vi "ReadDigitalLine.vi"(0 "device name":string="DAQ", 5 "port":i32, 7 "line":i32, 11 "error in":errorcluster) -> (4 "state":u8, 15 "error out":errorcluster)   [LabVIEW 2012]
uses:
  <vilib>/DAQmx/read.llb/DAQmx Read.vi
  <vilib>/DAQmx/read.llb/DAQmx Read (Digital Bool 1Line 1Point).vi
  <vilib>/DAQmx/create/channels.llb/DAQmx Create Channel (DI-Digital Input).vi
  <vilib>/DAQmx/miscellaneous.llb/DAQmx Fill In Error Info.vi
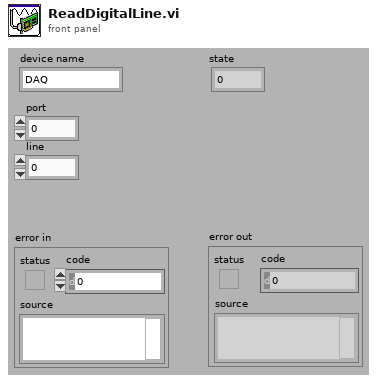
[diagram p1: front panel]
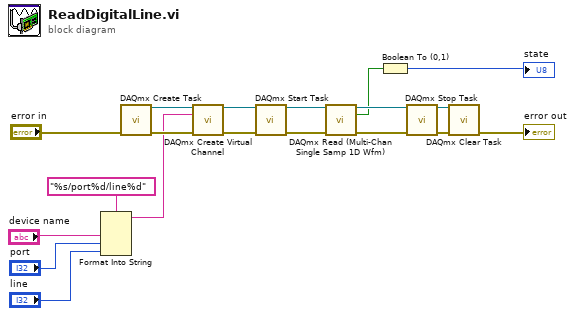
[diagram p0: block diagram]
diagram:
  n1 = Format Into String(format string="%s/port%d/line%d", "device name", "port", "line") -> (resulting string=w3:string)  [unwired: 2 in, 1 out]
  n2 = call <vilib>:"DAQmx Create Task.vi"("error in"="error in") -> ("task out"=w14:refnum<k21>, "error out"=w17:errorcluster)  [unwired: 13 in]
  n3 = call-poly <vilib>:"DAQmx Create Virtual Channel.vi"("task in"=w14, "lines"=w3, "error in"=w17) -> ("task out"=w12:refnum<k21>, "error out"=w13:errorcluster)  [unwired: 11 in]
  n4 = call <vilib>:"DAQmx Start Task.vi"("task/channels in"=w12, "error in"=w13) -> ("task out"=w9:refnum<k21>, "error out"=w16:errorcluster)  [unwired: 12 in]
  n5 = call-poly "DAQmx Read (Multi-Chan Single Samp 1D Wfm).vi"("task/channels in"=w9, "error in"=w16) -> ("task out"=w8:refnum<k21>, "data"=w2:bool, "error out"=w15:errorcluster)  [unwired: 11 in]
  n6 = Boolean To (0,1)(Boolean=w2) -> (0, 1=→"state":i16)
  n7 = call <vilib>:"DAQmx Stop Task.vi"("task/channels in"=w8, "error in"=w15) -> ("task out"=w10:refnum<k21>, "error out"=w11:errorcluster)  [unwired: 12 in]
  n8 = call <vilib>:"DAQmx Clear Task.vi"("task in"=w10, "error in"=w11) -> ("error out"=→"error out":errorcluster)  [unwired: 13 in]
